vi "Get Line Timing.vi"(8 "error in (no error)":errorcluster, 10 "Line index":i32, 11 "Master Device in":refnum<class "Master Device.lvclass">) -> (0 "error out":errorcluster, 2 "Line Timing":T1, 3 "Master Device out":refnum<class "Master Device.lvclass">)   [LabVIEW 2013, in "Master Device.lvclass"]
doc: "Stub to be overridden by Master child, e.g. PulseBlaster."
uses:
  Master Device.lvclass
  TypeDefs/LineTiming.ctl
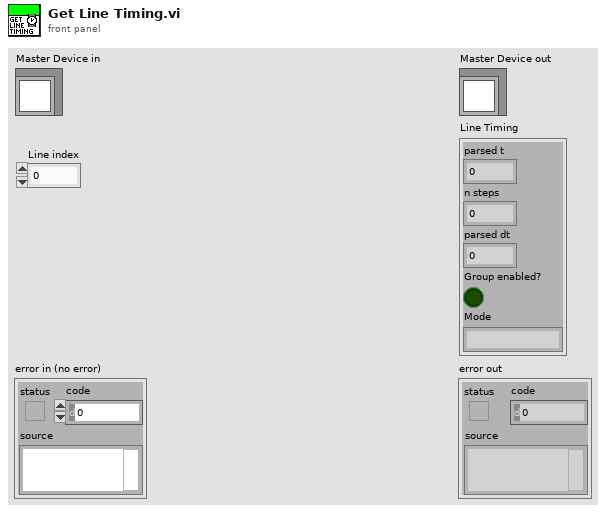
[diagram p1: front panel]
types:
  T1 = typedef "LineTiming.ctl" = cluster{"parsed t":dbl, "n steps":i32, "parsed dt":dbl, "Group enabled?":bool, "Mode":string}
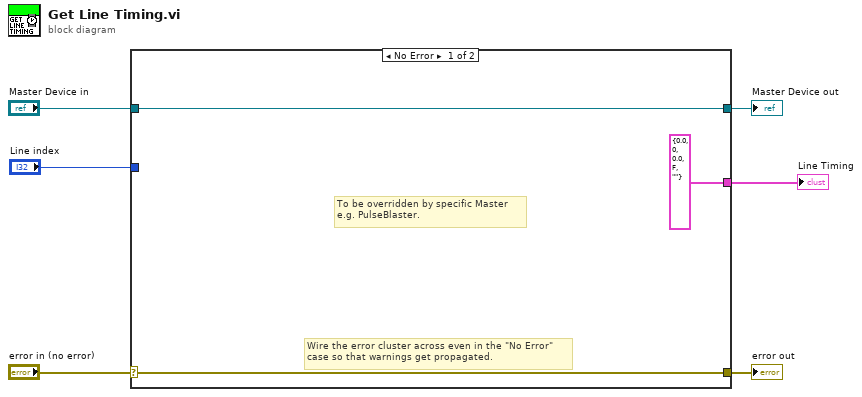
[diagram p0: block diagram]
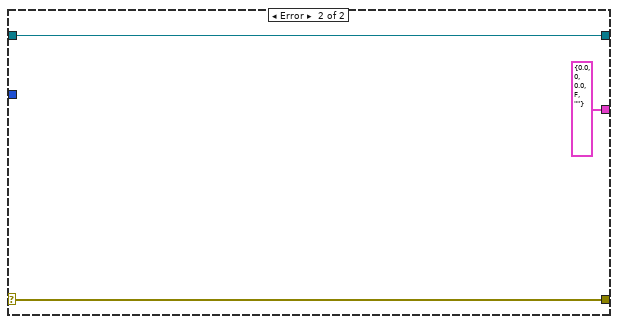
[diagram p2: hidden frame]
diagram:
  n1 = case shown="No Error" "error in (no error)" {
    selector: "error in (no error)" -> [w8 w12]
    tunnel: [w8 w12] -> w5
    tunnel: [w9 w11] -> w3
    tunnel: "Master Device in" -> [w9 w11]
    tunnel: "Line index" -> [_ _]
    tunnel: [T1 {"parsed t"=0.0, "n steps"=0, "parsed dt"=0.0, "Group enabled?"=FALSE, "Mode"=""} ("Line Timing") T1 {"parsed t"=0.0, "n steps"=0, "parsed dt"=0.0, "Group enabled?"=FALSE, "Mode"=""} ("Line Timing")] -> w1
    frame No Error {
      # "To be overridden by specific Master\ne.g. PulseBlaster."
      # "Wire the error cluster across even in the \"No Error\"\ncase so that warnings get propagated."
    }
    frame Error {
    }
  }
  "error out" <- w5
  "Master Device out" <- w3
  "Line Timing" <- w1
